vi "428 SCPI_Version 1.2.vi"(0 "VISA resource name":refnum<visa-resource-name>="COM5", 1 "baud rate":u32=9600, 4 "data bits":u16=8 min=5 max=8 step=1, 5 "parity":u16(ring) items=["None", "Odd", "Even", "Mark", "Space"], 7 "stop bits":u16(ring)=10 items=["1.0"=10, "1.5"=15, "2.0"=20], 15 "timeout (ms)":u32=5000, 21 "End read on termination character?":bool=TRUE, 24 "termination char\n(0xA = '\\n' = LF)":u8=10 format="%.0x", 25 "Input\nbuffer size":u32=4096) -> ()   [LabVIEW 2016]
doc: "The Advanced Serial Read and Write example performs a Serial Port Read, a Serial Port Write, or a combination of these actions while setting some advanced serial features like buffer size, termination characters, and XON/XOFF flow control. The user selects the actions (read or write) on the front panel. If both are selected, the VI will write the data first, read the data and then close the VISA session that is opened to the port. \n\nThe parameters set for the serial port must match the parameters of the connected instrument or device. In this example, the bytes to read parameter specifies the number of bytes that the serial port reads. If there were more bytes at the port than the number specified in bytes to read, those bytes would not be read. Also, if you specify to read more bytes than the number of bytes actually read, you might receive a timeout error message.\n\nINSTRUCTIONS:\n1) Select the serial resource and configuration parameters (baud rate, data bits, parity, stop bits, flow control).\n2) Termination character can be enabled and set. Also, set the required input buffer size prior to running the example.\n3) Select the operations to be performed. \n4) Connect the serial port to your device. If no device is available, perform a loopback test by doing one of the following. Short pins 2 and 3 on a RS-232 cable or short pin 4 to pin 8 and pin 5 to pin 9 on a RS-485/422 cable. \n5) Run the VI to see the data read. (The \"read string\" will match the \"string to write\" if a loopback test was performed.)\n\nThis example exposes several advanced features that you may need for your application. Not all applications need all the features shown in this example. The input buffer size is likely an important setting that you want to control in your application. This example expands upon the flow control option for XON and XOFF, allowing the user to choose those control characters. The timeout parameter has been brought to the front panel so a user can specify the time period the VISA Read will wait for the number of bytes to read before timing out. Also, the user has several controls for the termination character, which is discussed later.\n\nNote that you can press the write and read buttons and change the bytes to read parameters on the fly, while the example is running. However, you must stop the example to change the other configuration parameters after the example has started running, and then run again.\n\nSet the I/O buffer size slightly higher the amount of data you expect to receive. This is very important for applications that don't use flow control, as you may lose characters if the receive buffer overflows.\n\nSetting the timeout period ensures that the operation returns with a timeout error if the operation cannot be performed in the specified time period. \n\nSome devices require a termination character in order to identify the end of command strings. Some devices send a termination character to signify the end of data to be read. \n\nThis example shows how you can end the Read operation once a termination character is detected in the buffer and/or append a termination character at the end of the Write data. To enable the Read to end on a termination character, use the VISA Configure Serial Port or use the VISA Properties Serial End Mode for Reads, Termination Character Enable, and Termination Character. To end the Write with a termination character, use the VISA Properties Serial End Mode for Writes, the Send End Enable, and Termination Character. In this example, the same termination character is used for both the Read and the Write. You can specify two different characters for your application, if desired.\n\nYour application may require specific characters for the XON/XOFF Flow Control. You can specify these characters with the VISA Properties Flow Control XOFF Character and Flow Control XON Character. Note that if the standard XON and XOFF characters are used, then decimal 17 and 19 are unavailable for data values. Remember that using flow control and setting an adequate buffer size allow you to prevent buffer overflows."
panel:
  in  "Measurement Type":enum16{"Measure", "Read", "Fetch"}(ring)
  out "Input string 2":string=":MEAS:SCAL:WAV?"
  in  "Measurement Command":T1(ring)=enum."Wavelength"
  in  "Response Format":enum16{"Scalar", "Array"}(ring)
  in  "Loop Time Delay (ms)":u32=1000
  out "Data Out":string="1552.2096\r\n"
  in  "bytes to read":u32=1500
  out "actual bytes read":u32=11
  in  "flow control":u16(ring) items=["None", "On"]
  out "Loop Count":i32=21
  in  "Log File Path":path=path "C:/Documents and Settings/BillG/Desktop/Temp/428_10GHzFSR.txt"
  in  "Stop":bool
  in  "End write with termination character?":bool=TRUE
  # "428 SCPI Example"
  # "Select the serial resource and the operations to be performed. The VI will write the Input string first, read data,  loop until the STOP button is pressed, and then close the VISA session that is opened to the port.  This VI will wait until the specified number of bytes is received at the port until the timeout period is met.  Only the specified number of bytes will be read unless the read ends on a termination character.  The termination character can be enabled and set.  Also, set the required input buffer size prior to running the example."
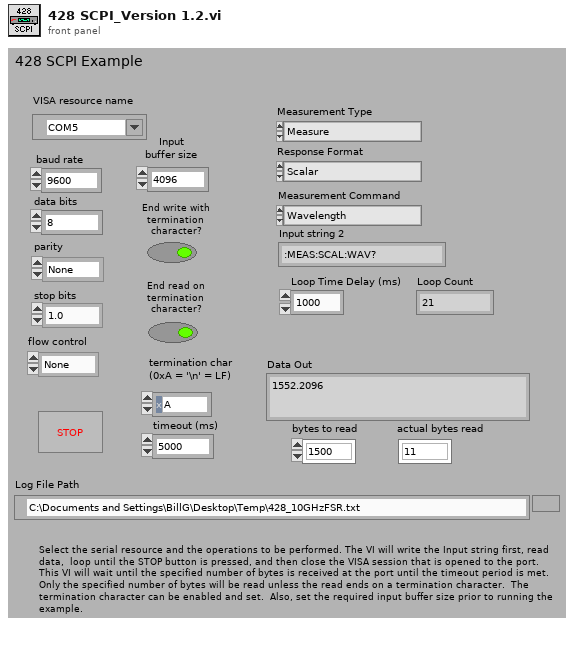
[diagram p1: front panel]
types:
  T1 = enum16{"Power", "Environment", "Wavelength", "Wave Number", "Frequency"}
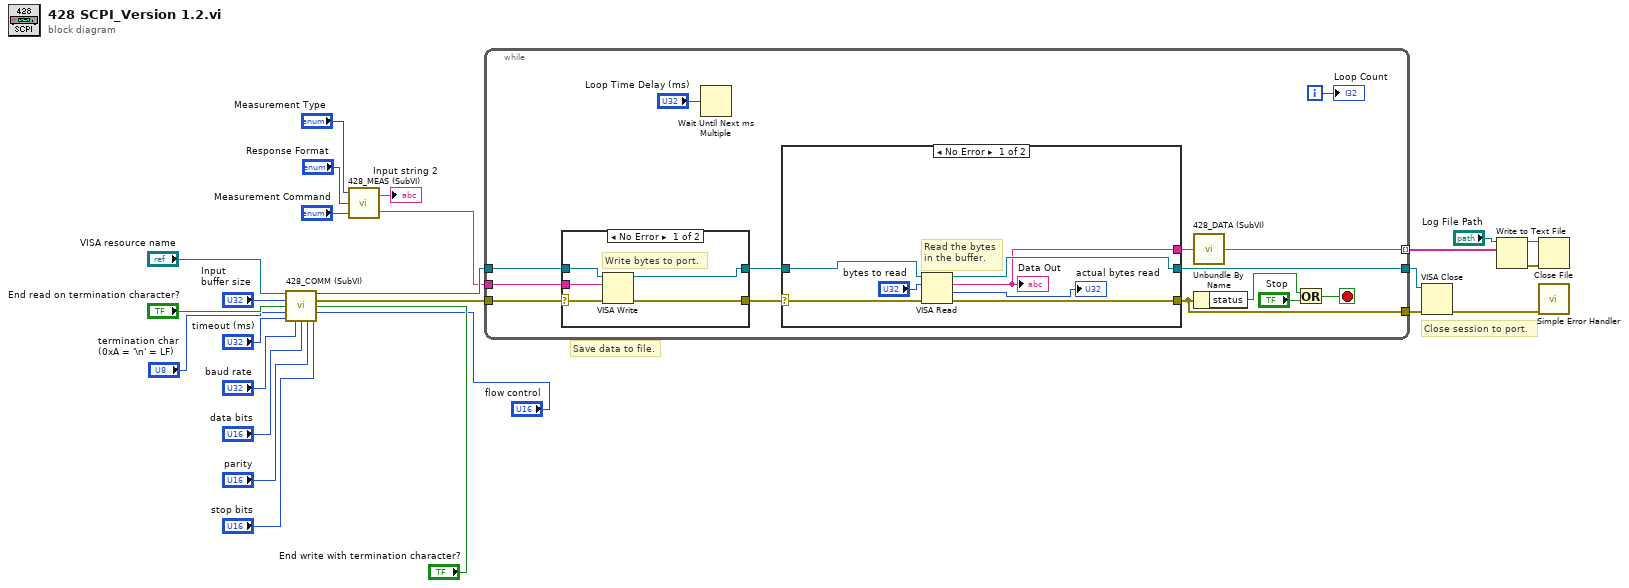
[diagram p0: block diagram]
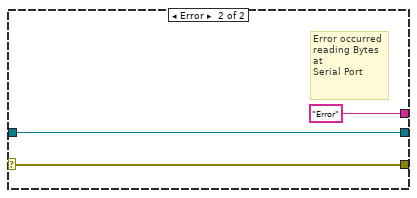
[diagram p2: hidden frame]
diagram:
  # "Save data to file."
  # "Close session to port."
  n1 = call "428_COMM (SubVI).vi"("VISA resource name"="VISA resource name", "Input\nbuffer size"="Input\nbuffer size", "End read on termination character?"="End read on termination character?", "End write with termination character?"="End write with termination character?", "termination char\n(0xA = '\\n' = LF)"="termination char\n(0xA = '\\n' = LF)", "flow control"="flow control", "timeout (ms)"="timeout (ms)", "baud rate"="baud rate", "data bits"="data bits", "parity"="parity", "stop bits"="stop bits") -> ("VISA resource name out"=w8:refnum<visa-resource-name>, "error out"=w7:errorcluster)  [unwired: 3 in]
  n2 = call "428_MEAS (SubVI).vi"("Measurement Command"="Measurement Command", "Response Format"="Response Format", "Measurement Type"="Measurement Type") -> ("String"=w2:string, "Input string 2"=→"Input string 2":string)
  n3 = while {
    tunnel: w7 -> [w31]
    tunnel: w8 -> [w32]
    tunnel: [w28] -> w14
    tunnel: [w27] -> w9
    tunnel: w2 -> [w33]
    tunnel: [w35] -> w12 mode=indexing
    i -> [w36]
    stop <- w38 stop-if-true
    n4 = case shown="No Error" w31 {
      selector: w31 -> [w51 w56]
      tunnel: [w54 w55] -> w30
      tunnel: [w53 w56] -> w29
      tunnel: w32 -> [w52 w55]
      tunnel: w33 -> [w50 _]
      frame No Error {
        # "Write bytes to port."
        n5 = VISA Write(VISA resource name=w52, write buffer=w50, error in (no error)=w51) -> (VISA resource name out=w54:refnum<visa-resource-name>, error out=w53:errorcluster)  [unwired: 1 out]
      }
      frame Error {
      }
    }
    n6 = Wait Until Next ms Multiple(millisecond multiple="Loop Time Delay (ms)") -> ()  [unwired: 1 out]
    n7 = case "Read bytes from port." shown="No Error" w29 {
      selector: w29 -> [w42 w48]
      tunnel: [w45 w48] -> w27
      tunnel: [w46 w49] -> w28
      tunnel: w30 -> [w43 w49]
      tunnel: [w40 "Error"] -> w26
      frame No Error {
        # "Read the bytes\nin the buffer."
        n8 = VISA Read(VISA resource name=w43, byte count="bytes to read", error in (no error)=w42) -> (VISA resource name out=w46:refnum<visa-resource-name>, read buffer=w40:string, return count=→"actual bytes read":u32, error out=w45:errorcluster)
        "Data Out" <- w40
      }
      frame Error {
        # "Error occurred \nreading Bytes at \nSerial Port"
      }
    }
    n9 = call "428_DATA (SubVI).vi"("read buffer"=w26) -> ("trimmed string"=w35:string)
    n10 = Unbundle By Name(w27) -> ("status"=w39:bool)
    n11 = Or(x=w39, y="Stop") -> (x .or. y?=w38:bool)
    "Loop Count" <- w36
  }
  n12 = VISA Close(VISA resource name=w14, error in (no error)=w9) -> (error out=w23:errorcluster)
  n13 = Write to Text File(file (use dialog)="Log File Path", text=w12) -> (refnum out=w11:refnum<file>, error out=w10:errorcluster)  [unwired: 2 in, 1 out]
  n14 = Close File(refnum=w11, error in=w10) -> ()  [unwired: 2 out]
  n15 = call <vilib>:"Simple Error Handler.vi"("error in (no error)"=w23) -> ()  [unwired: 4 in, 5 out]
